vi "AD2_WFG_SDK_Init.vi"(0 "object in":refnum<class "AD2_WFG_SDK.lvclass">, 2 "phdwf":i32, 5 "error in (no error)":errorcluster) -> (14 "object out":refnum<class "AD2_WFG_SDK.lvclass">, 19 "error out":errorcluster)   [LabVIEW 2021, in "AD2_WFG_SDK.lvclass"]
uses:
  AD2_WFG_SDK.lvclass
  AD2_WFG_SDK.lvclass/AD2_WFG_SDK.ctl
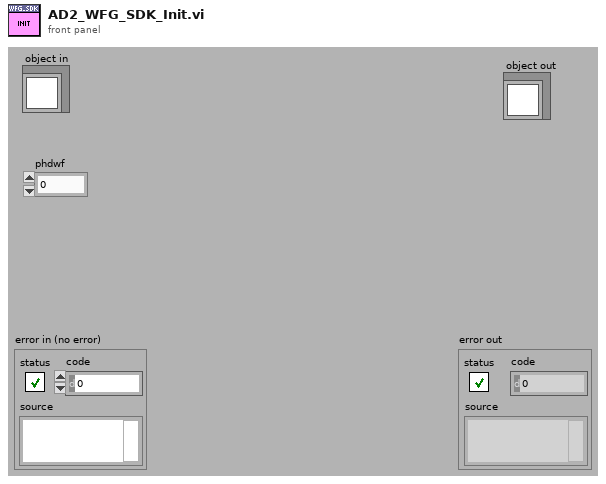
[diagram p1: front panel]
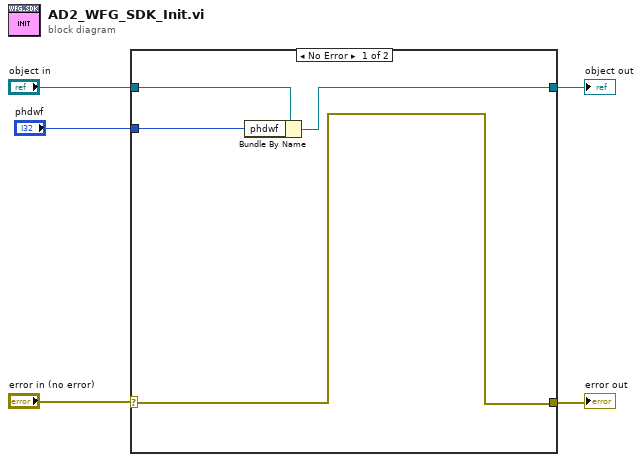
[diagram p0: block diagram]
diagram:
  n1 = case shown="No Error" "error in (no error)" {
    selector: "error in (no error)" -> [w8 w10]
    tunnel: "object in" -> [w9 w11]
    tunnel: [w7 w11] -> w4
    tunnel: [w8 w10] -> w2
    tunnel: "phdwf" -> [w6 _]
    frame No Error {
      n2 = Bundle By Name(cluster=w9, "phdwf"=w6) -> (w7:refnum<class "AD2_WFG_SDK.lvclass">)
    }
    frame Error {
    }
  }
  "object out" <- w4
  "error out" <- w2
